vi "myRIO_Read.vi"(8 "error in":errorcluster, 10 "AI Ref In":T1, 11 "I2C Ref Out in":T10) -> (0 "error out":errorcluster, 1 "Data":dbl[](array[numeric]), 2 "AI Ref Out":T1, 3 "I2C Ref Out out":T10)   [LabVIEW 2019]
uses:
  <vilib>/myRIO/Instrument Drivers/Onboard IO/I2C/typedefs/I2C Reference.ctl
  <vilib>/myRIO/Common/Instrument Driver Framework/Utilities/typedefs/myRIO Generic Hardware Reference.ctl
  <vilib>/myRIO/Common/Instrument Driver Framework/Utilities/typedefs/Hardware Version Enum.ctl
  <vilib>/myRIO/Common/Instrument Driver Framework/Utilities/typedefs/myRIO v1.0 Reference.ctl
  <vilib>/myRIO/Common/Instrument Driver Framework/Utilities/typedefs/Generic FPGA Reference.ctl
  <vilib>/myRIO/Common/Instrument Driver Framework/myRIO v1.0/I2C/typedefs/I2C Channels Enum.ctl
  <vilib>/myRIO/Instrument Drivers/Onboard IO/I2C/typedefs/I2C Configuration.ctl
  <vilib>/myRIO/Instrument Drivers/Onboard IO/I2C/typedefs/I2C Transfer Rate.ctl
  <vilib>/myRIO/Instrument Drivers/Onboard IO/AI/typedefs/AI Reference.ctl
  <vilib>/myRIO/Common/Instrument Driver Framework/myRIO v1.0/AI/typedefs/AI Channels List.ctl
  <vilib>/myRIO/Common/Instrument Driver Framework/myRIO v1.0/AI/typedefs/AI Channels Enum.ctl
  <vilib>/myRIO/Common/Instrument Driver Framework/Utilities/typedefs/Analog Scaling Constants List.ctl
  <vilib>/myRIO/Common/Instrument Driver Framework/Utilities/typedefs/Analog Scaling Constants.ctl
  TypeDef/#TypeDef_EnumSensorConnection.ctl
  <vilib>/Utility/error.llb/Error Cluster From Error Code.vi
  <vilib>/myRIO/Common/Instrument Driver Framework/myRIO v1.0/AI/vis/myRIO v1.0 Read AI.vi
  <vilib>/myRIO/Common/Instrument Driver Framework/myRIO v1.0/I2C/vis/myRIO v1.0 Write I2C.vi
  <vilib>/myRIO/Common/Instrument Driver Framework/myRIO v1.0/I2C/vis/myRIO v1.0 Read I2C.vi
  <vilib>/myRIO/Instrument Drivers/Onboard IO/I2C/I2C.lvlib
  <vilib>/myRIO/Instrument Drivers/Onboard IO/AI/AI.lvlib
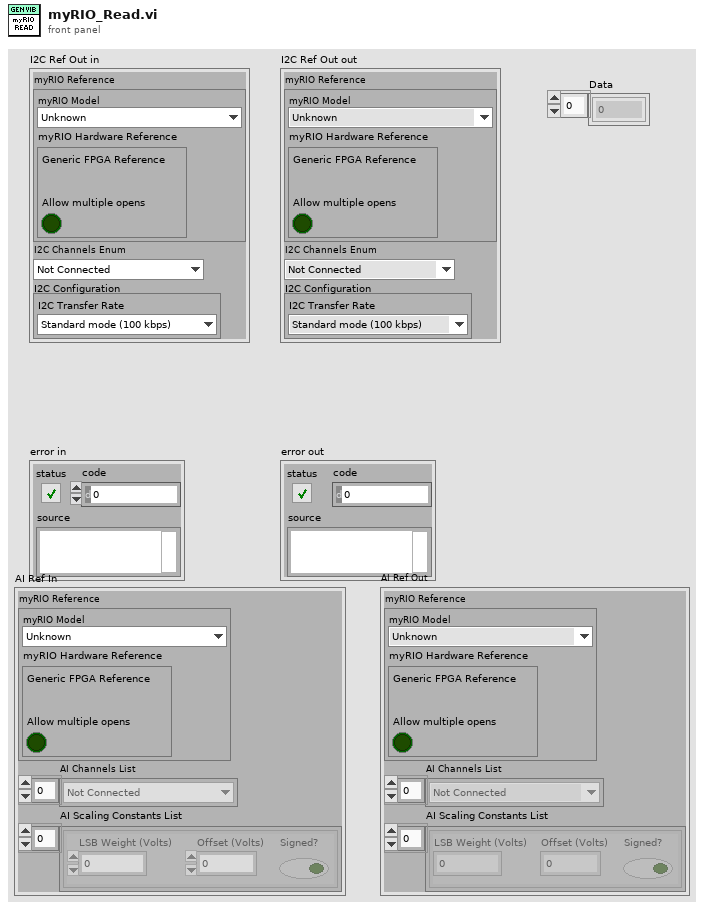
[diagram p1: front panel]
types:
  T1 = typedef "AI.lvlib/AI Reference.ctl" = cluster{"myRIO Reference":T2, "AI Channels List":T6, "AI Scaling Constants List":T8}
  T2 = typedef "myRIO Generic Hardware Reference.ctl" = cluster{"myRIO Model":T3, "myRIO Hardware Reference":T4}
  T3 = typedef "Hardware Version Enum.ctl" = enum16{"Unknown", "myRIO-1900", "myRIO-1950", "roboRIO", "NI ELVIS RIO CM", "ELVIS III"}
  T4 = typedef "myRIO v1.0 Reference.ctl" = cluster{"Generic FPGA Reference":T5, "Allow multiple opens":bool}
  T5 = typedef "Generic FPGA Reference.ctl" = refnum<k20>
  T6 = typedef "AI Channels List.ctl" = T7[]
  T7 = typedef "AI Channels Enum.ctl" = enum16{"Not Connected", "AudioIn/Left", "AudioIn/Right", "C/AI0", "C/AI1", "A/AI0", "A/AI1", "A/AI2", "A/AI3", "A/AI4", "A/AI5", "A/AI6", "A/AI7", "B/AI0", "B/AI1", "B/AI2", "B/AI3", "B/AI4", "B/AI5", "B/AI6", "B/AI7", "AI/AI0", "AI/AI1", "AI/AI2", "AI/AI3", "A/AI0 (DIFF)", "A/AI1 (DIFF)", "A/AI2 (DIFF)", "A/AI3 (DIFF)", "B/AI0 (DIFF)", "B/AI1 (DIFF)", "B/AI2 (DIFF)", "B/AI3 (DIFF)"}
  T8 = typedef "Analog Scaling Constants List.ctl" = T9[]
  T9 = typedef "Analog Scaling Constants.ctl" = cluster{"LSB Weight (Volts)":dbl, "Offset (Volts)":dbl, "Signed?":bool}
  T10 = typedef "I2C.lvlib/I2C Reference.ctl" = cluster{"myRIO Reference":T2, "I2C Channels Enum":T11, "I2C Configuration":T12}
  T11 = typedef "I2C Channels Enum.ctl" = enum16{"Not Connected", "A/I2C", "B/I2C", "I2C/I2C"}
  T12 = typedef "I2C.lvlib/I2C Configuration.ctl" = cluster{"I2C Transfer Rate":T13}
  T13 = typedef "I2C.lvlib/I2C Transfer Rate.ctl" = enum16{"Standard mode (100 kbps)", "Fast mode (400 kbps)"}
  T14 = typedef "#TypeDef_EnumSensorConnection.ctl" = enum16{"Analog", "Digital"}
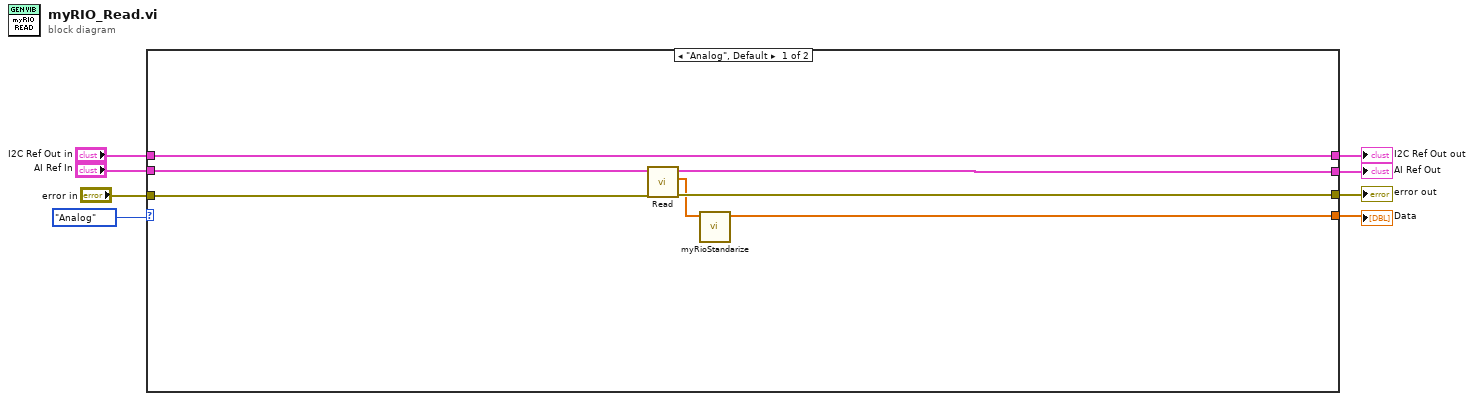
[diagram p0: block diagram]
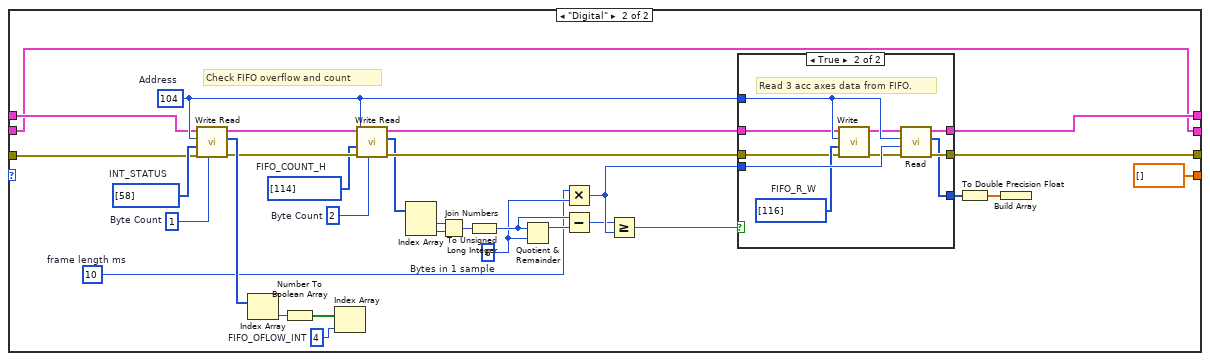
[diagram p2: hidden frame]
diagram:
  n1 = case shown="\"Analog\", Default" #TypeDef_EnumSensorConnection."Analog" {
    tunnel: [w12 w45] -> w8
    tunnel: [w11 w44] -> w7
    tunnel: "error in" -> [w15 w20]
    tunnel: "I2C Ref Out in" -> [w12 w19]
    tunnel: "AI Ref In" -> [w14 w17]
    tunnel: [w13 w17] -> w2
    tunnel: [w9 dbl[] [] ("Values")] -> w1
    frame "Analog", Default {
      n2 = call <vilib>:"Read.vi"("error in (no error)"=w15, "AI Ref In"=w14) -> ("error out"=w11:errorcluster, "Values"=w10:dbl[], "AI Ref Out"=w13:T1)  [unwired: 7 in]
      n3 = call "myRioStandarize.vi"("Data in"=w10) -> ("Data out"=w9:dbl[])  [unwired: 10 in]
    }
    frame "Digital" {
      w21 = i64 10  # frame length ms
      w32 = 4  # FIFO_OFLOW_INT
      w29 = u32 1  # Byte Count
      w28 = u8[] [58]  # INT_STATUS
      w38 = u32 6  # Bytes in 1 sample
      w23 = u8[] [114]  # FIFO_COUNT_H
      w37 = u8 104  # Address
      w22 = u32 2  # Byte Count
      # "Check FIFO overflow and count"
      n4 = call <vilib>:"Write Read.vi"("Byte Count"=w29, "error in (no error)"=w20, "Bytes to Write"=w28, "Slave Address (7-bit)"=w37, "I2C Ref In"=w19) -> ("error out"=w27:errorcluster, "Bytes Read"=w33:u8[], "I2C Ref Out"=w26:T10)  [unwired: 3 in]
      n5 = Index Array(array=w33) -> (element=w30:u8)  [unwired: 1 in]
      n6 = Number To Boolean Array(number=w30) -> (Boolean array=w31:bool[])
      n7 = Index Array(array=w31, index=w32) -> ()  [unwired: 1 out]
      n8 = call <vilib>:"Write Read.vi"("Byte Count"=w22, "error in (no error)"=w27, "Bytes to Write"=w23, "Slave Address (7-bit)"=w37, "I2C Ref In"=w26) -> ("error out"=w41:errorcluster, "Bytes Read"=w24:u8[], "I2C Ref Out"=w18:T10)  [unwired: 3 in]
      n9 = Index Array(array=w24) -> (element #1=w25:u8, element #2=w36:u8)  [unwired: 2 in]
      n10 = Join Numbers(hi=w25, lo=w36) -> ((hi.lo)=w35:u16)
      n11 = To Unsigned Long Integer(number=w35) -> (unsigned 32bit integer=w42:u32)
      n12 = Quotient & Remainder(x=w42, y=w38) -> (x-y*floor(x/y)=w34:u32)  [unwired: 1 out]
      n13 = Multiply(x=w21, y=w38) -> (x*y=w40:i64)
      n14 = Subtract(x=w42, y=w34) -> (x-y=w39:u32)
      n15 = Greater Or Equal?(x=w39, y=w40) -> (x >= y?=w43:bool)
      n16 = case shown="True" w43 {
        tunnel: [w49 w52] -> w44
        tunnel: w37 -> [_ w56]
        tunnel: w41 -> [w49 w57]
        tunnel: w40 -> [_ w59]
        tunnel: w18 -> [w48 w55]
        tunnel: [w48 w51] -> w45
        tunnel: [_ w50] -> w46
        frame False {
        }
        frame True {
          w58 = u8[] [116]  # FIFO_R_W
          # "Read 3 acc axes data from FIFO."
          n17 = call <vilib>:"Write.vi"("error in (no error)"=w57, "Bytes to Write"=w58, "Slave Address (7-bit)"=w56, "I2C Ref In"=w55) -> ("error out"=w54:errorcluster, "I2C Ref Out"=w53:T10)  [unwired: 6 in]
          n18 = call <vilib>:"Read.vi"("error in (no error)"=w54, "Byte Count"=w59, "Slave Address (7-bit)"=w56, "I2C Ref In"=w53) -> ("error out"=w52:errorcluster, "Bytes Read"=w50:u8[], "I2C Ref Out"=w51:T10)  [unwired: 4 in]
        }
      }
      n19 = To Double Precision Float(number=w46) -> (double precision float=w47:dbl[])
      n20 = Build Array(w47) -> ()  [unwired: 1 out]
    }
  }
  "I2C Ref Out out" <- w8
  "error out" <- w7
  "AI Ref Out" <- w2
  "Data" <- w1
